vi "Export results.vi"(7 "Pixel size (nm)":dbl, 8 "error in (no error)":errorcluster, 9 "Template Image":T2, 10 "Directory with images":path, 11 "Results":T1[](array[typedef]) {"Raw matches"."Bounding Box"."y" format="%.2f"; "Raw matches"."Bounding Box"."x" format="%.2f"; "Raw matches"."Position"."y" format="%.2f"; "Raw matches"."Position"."x" format="%.2f"; "Raw matches"."Score" format="%.2f"; "Raw matches"."Scale" format="%.2f"; "Raw matches"."Angle" format="%.2f"}) -> (0 "error out":errorcluster, 2 "Created results dir":path)   [LabVIEW 2011]
uses:
  <vilib>/vision/Image Controls.llb/IMAQ Image.ctl
  Worker result.ctl
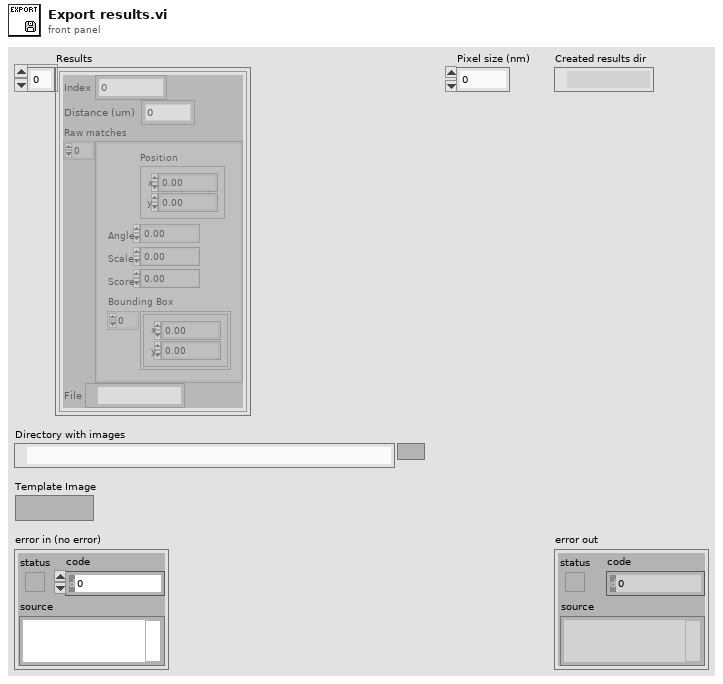
[diagram p1: front panel]
types:
  T1 = typedef "Worker result.ctl" = cluster{"Index":u32, "Distance (um)":dbl, "Raw matches":cluster{"Position":cluster{"x":sgl, "y":sgl}, "Angle":sgl, "Scale":sgl, "Score":sgl, "Bounding Box":cluster{"x":sgl, "y":sgl}[]}[], "File":path}
  T2 = typedef "IMAQ Image.ctl" = refnum<image>
  T3 = cluster{"Position":cluster{"x":sgl, "y":sgl}, "Angle":sgl, "Scale":sgl, "Score":sgl, "Bounding Box":cluster{"x":sgl, "y":sgl}[]}[]
  T4 = cluster{"Position":cluster{"x":sgl, "y":sgl}, "Angle":sgl, "Scale":sgl, "Score":sgl, "Bounding Box":cluster{"x":sgl, "y":sgl}[]}
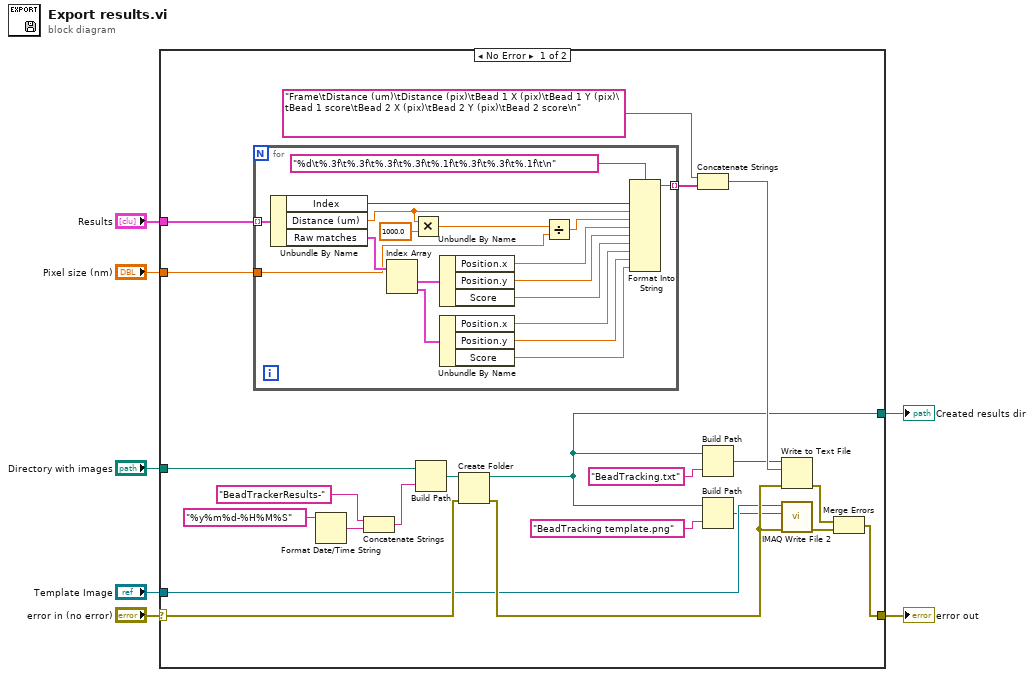
[diagram p0: block diagram]
diagram:
  n1 = case shown="No Error" "error in (no error)" {
    selector: "error in (no error)" -> [w26 w48]
    tunnel: "Template Image" -> [w24 _]
    tunnel: "Directory with images" -> [w14 _]
    tunnel: "Results" -> [w16 _]
    tunnel: "Pixel size (nm)" -> [w15 _]
    tunnel: [w27 w48] -> w7
    tunnel: [w8 _] -> w1
    frame No Error {
      n2 = for {
        tunnel: w16 -> [w47] mode=indexing
        tunnel: [w35] -> w17 mode=indexing
        tunnel: w15 -> [w30]
        n3 = Unbundle By Name(w47) -> ("Index"=w43:u32, "Distance (um)"=w32:dbl, "Raw matches"=w46:T3)
        n4 = Index Array(array=w46) -> (element #1=w45:T4, element #2=w44:T4)  [unwired: 2 in]
        n5 = Multiply(x=w32, y=1000.0) -> (x*y=w33:dbl)
        n6 = Unbundle By Name(w45) -> ("Position.x"=w42:sgl, "Position.y"=w41:sgl, "Score"=w40:sgl)
        n7 = Unbundle By Name(w44) -> ("Position.x"=w39:sgl, "Position.y"=w38:sgl, "Score"=w37:sgl)
        n8 = Divide(x=w33, y=w30) -> (x/y=w31:dbl)
        n9 = Format Into String(format string="%d\t%.3f\t%.3f\t%.3f\t%.3f\t%.1f\t%.3f\t%.3f\t%.1f\t\n", w43, w32, w31, w42, w41, w40, w39, w38, w37) -> (resulting string=w35:string)  [unwired: 2 in, 1 out]
      }
      n10 = Format Date/Time String(time format string (%c)="%y%m%d-%H%M%S") -> (date/time string=w12:string)  [unwired: 2 in]
      n11 = Concatenate Strings("BeadTrackerResults-", w12) -> (w10:string)
      n12 = Build Path(base path=w14, name or relative path=w10) -> (appended path=w9:path)
      n13 = Create Folder(path (use dialog)=w9, error in=w26) -> (created path=w8:path, error out=w25:errorcluster)  [unwired: 1 in, 1 out]
      n14 = Concatenate Strings("Frame\tDistance (um)\tDistance (pix)\tBead 1 X (pix)\tBead 1 Y (pix)\tBead 1 score\tBead 2 X (pix)\tBead 2 Y (pix)\tBead 2 score\n" ("format string"), w17) -> (w21:string)
      n15 = Build Path(base path=w8, name or relative path="BeadTracking.txt") -> (appended path=w20:path)
      n16 = Build Path(base path=w8, name or relative path="BeadTracking template.png") -> (appended path=w23:path)
      n17 = Write to Text File(file (use dialog)=w20, text=w21, error in=w25) -> (error out=w28:errorcluster)  [unwired: 1 in, 2 out]
      n18 = call-poly "IMAQ Write File 2"("error in (no error)"=w25, "File Path"=w23, "Image"=w24) -> ("error out"=w29:errorcluster)  [unwired: 7 in, 1 out]
      n19 = Merge Errors(w28, w29) -> (w27:errorcluster)
    }
    frame Error {
    }
  }
  "error out" <- w7
  "Created results dir" <- w1
